vi "Handle Error.vi"(8 "error in (no error)":errorcluster, 11 "Client Controller in":refnum<class "Client Controller.lvclass">) -> (0 "error out":errorcluster, 2 "stop actor?":bool=TRUE, 3 "Client Controller out":refnum<class "Client Controller.lvclass">)   [LabVIEW 2013, in "Client Controller.lvlib" / "Client Controller.lvclass"]
doc: "(<B>Filename</B>: Actor Framework.lvlib:Actor.lvclass:Handle Error.vi)\n\nDefines how the actor handles an error that occurred while processing a message.\n\nBy default, this method does nothing except stop the actor. This method also treats error code 43 (coming from <B>error in</B>) as a sign that the actor shut down normally. In this situation, the Handle Error method does not return the error on <B>error out</B>, meaning the actor's caller will not receive it. All other error codes will be returned on <B>error out</B>.\n\nA descendant class may override this method to change this behavior."
uses:
  Client Controller.lvclass
  Msmt-Framework/user.lib/Common Components/Controller/Controller.lvclass
  Client Controller.lvclass/Client Controller.ctl
  <vilib>/ActorFramework/Actor/Actor.lvclass/Actor.ctl
  <vilib>/ActorFramework/Message Enqueuer/Message Enqueuer.lvclass/Message Enqueuer.ctl
  <vilib>/ActorFramework/Message Enqueuer/Init from Existing Queue.vi
  <vilib>/ActorFramework/Message Enqueuer/Enqueue.vi
  <vilib>/ActorFramework/Message Priority Queue/Priority Enqueue.vi
  <vilib>/ActorFramework/Message Enqueuer/Message Enqueuer.lvclass
  Messages/Negotiate Server Connection Msg/Negotiate Server Connection Msg.lvclass
  <vilib>/ActorFramework/Actor/Actor.lvclass
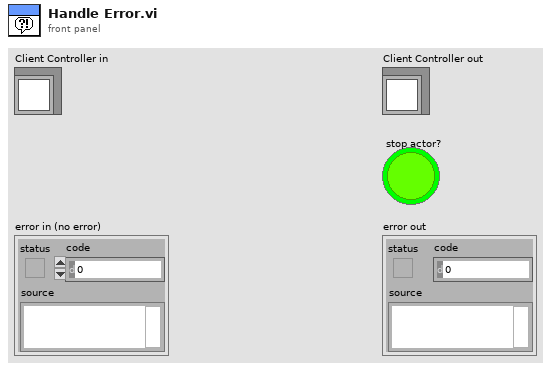
[diagram p1: front panel]
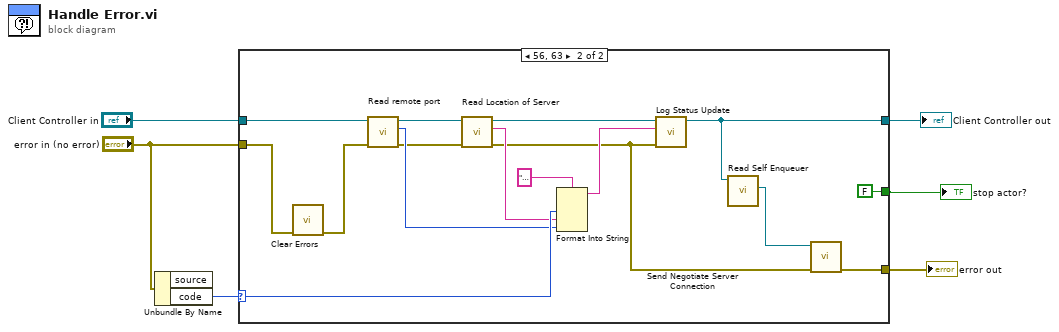
[diagram p0: block diagram]
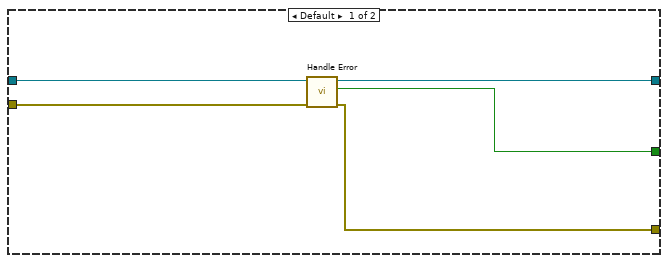
[diagram p2: hidden frame]
diagram:
  n1 = Unbundle By Name("error in (no error)") -> ("code"=w6:i32)  [unwired: 1 out]
  n2 = case shown="56, 63" w6 {
    selector: w6 -> [_ w26]
    tunnel: "Client Controller in" -> [w11 w23]
    tunnel: "error in (no error)" -> [w10 w16]
    tunnel: [w9 w18] -> w2
    tunnel: [w8 w14] -> w1
    tunnel: [w7 FALSE ("stop actor?")] -> w3
    frame Default {
      n3 = call-parent "Handle Error.vi"("error in (no error)"=w10, "Controller in"=w11) -> ("error out"=w8:errorcluster, "stop actor?"=w7:bool, "Controller out"=w9:refnum<class "Client Controller.lvclass">)  [unwired: 7 in]
    }
    frame 56, 63 {
      n4 = call <vilib>:"Clear Errors.vi"("error in (no error)"=w16) -> ("error out"=w15:errorcluster)  [unwired: 6 in]
      n5 = call "Read remote port.vi"("error in (no error)"=w15, "Client Controller in"=w23) -> ("error out"=w20:errorcluster, "remote port"=w24:u16, "Client Controller out"=w22:refnum<class "Client Controller.lvclass">)  [unwired: 7 in]
      n6 = call "Read Location of Server.vi"("error in (no error)"=w20, "Client Controller in"=w22) -> ("error out"=w12:errorcluster, "Location of Server"=w25:string, "Client Controller out"=w21:refnum<class "Client Controller.lvclass">)  [unwired: 7 in]
      n7 = Format Into String(format string="ERROR %d: Cannot connect to server %s:%d", w26, w25, w24) -> (resulting string=w19:string)  [unwired: 2 in, 1 out]
      n8 = call-dynamic "Log Status Update.vi"("error in (no error)"=w12, "String"=w19, "Controller in"=w21) -> ("Controller out"=w18:refnum<class "Client Controller.lvclass">)  [unwired: 7 in, 1 out]
      n9 = call <vilib>:"Read Self Enqueuer.vi"("Actor"=w18) -> ("Self Enqueuer"=w17:refnum<class "Message Enqueuer.lvclass">)  [unwired: 10 in]
      n10 = call "Send Negotiate Server Connection.vi"("error in (no error)"=w12, "Message Enqueuer"=w17) -> ("error out"=w14:errorcluster)  [unwired: 8 in, 1 out]
    }
  }
  "Client Controller out" <- w2
  "error out" <- w1
  "stop actor?" <- w3
